vi "MoveJogStep.vi"(8 "Error In":errorcluster, 10 "direction":i32(ring)=1 items=["Forward"=1, "Backward"=2], 11 "Thorlabs In":refnum<class "Thorlabs.lvclass">) -> (0 "Error Out":errorcluster, 3 "Thorlabs Out":refnum<class "Thorlabs.lvclass">)   [LabVIEW 2018, in "Thorlabs.lvlib" / "Thorlabs.lvclass"]
doc: "Moves the Axis by a the step size for the job parameters. This is done in the direction specified.\n\nCreator: Slade Jeppesen\nCreated Date: 10/02/20"
uses:
  Thorlabs.lvclass
  Thorlabs.lvclass/Thorlabs.ctl
  C:/AME Test Engineering/LabVIEW/PPLs/Axis/DLLs/ThorLabs.MotionControl.KCube.DCServoCLI.dll
  PPLs/Axis/DLLs/ThorLabs.MotionControl.KCube.DCServoCLI.dll
  31825a4c-c9b7-413c-8d5f-0f6836adbe55.vi
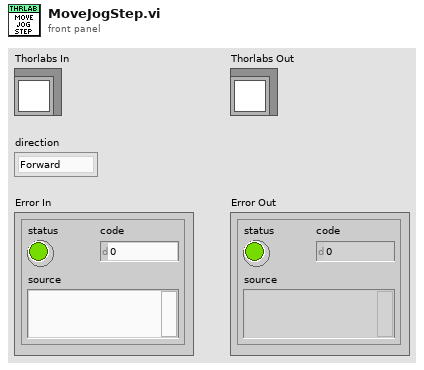
[diagram p1: front panel]
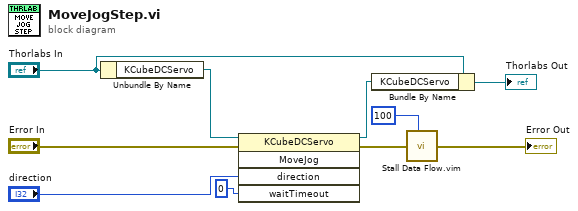
[diagram p0: block diagram]
diagram:
  n1 = Unbundle By Name("Thorlabs In") -> ("KCubeDCServo"=w10:refnum<k24>)
  n2 = invoke class="KCubeDCServo" method="MoveJog"(reference=w10, error in="Error In", "direction"="direction", "waitTimeout"=0) -> (reference out=w5:refnum<k24>, error out=w3:errorcluster)  [unwired: 1 in, 3 out]
  n3 = Bundle By Name(cluster="Thorlabs In", "KCubeDCServo"=w5) -> (→"Thorlabs Out":refnum<class "Thorlabs.lvclass">)
  n4 = call "Stall Data Flow.vim"("value in"=w3, "milliseconds to wait"=u32 100) -> ("value out"=→"Error Out":errorcluster)  [unwired: 1 out]
